vi "Fast_sequence_update_slot.vi"(1 "FPGA Ref":T1, 2 "Points":cluster{string, "data":u64, "data":dbl}, 3 "Inst param":T2) -> (0 "FPGA Ref Out":T1)   [LabVIEW 2013]
uses:
  fpga-bitfile-ref.ctl
  sequence slot/slot-use.ctl
  sequence slot/triggers.ctl
  sequence slot/DAC.ctl
  sequence slot/DAC_fastseq-offset.ctl
  sequence slot/timing.ctl
  sequence slot/jump.ctl
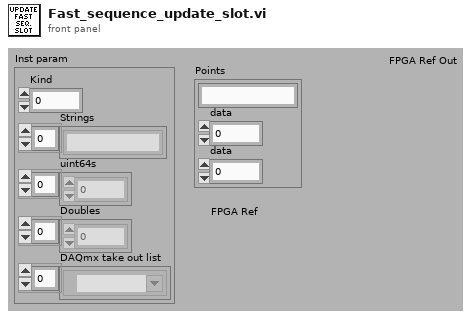
[diagram p1: front panel]
types:
  T1 = typedef "fpga-bitfile-ref.ctl" = refnum<k20>
  T2 = cluster{"Kind":u16, "Strings":string[], "uint64s":u64[], "Doubles":dbl[], "DAQmx take out list":refnum<k21>[]}
  T3 = typedef "slot-use.ctl" = enum8{"DAC", "timing", "triggers", "jump"}
  T4 = typedef "triggers.ctl" = cluster{"triggers":cluster{"1":bool, "2":bool, "3":bool, "4":bool}, "stop":bool}
  T5 = typedef "DAC.ctl" = cluster{"FastChanNum":u8, "DAC offset":T6}
  T6 = typedef "DAC_fastseq-offset.ctl" = sgl
  T7 = typedef "timing.ctl" = sgl
  T8 = typedef "jump.ctl" = u16
  T9 = cluster{"use":T3, "Triggers":T4, "DAC":T5, "timing":T7, "slot#":T8}
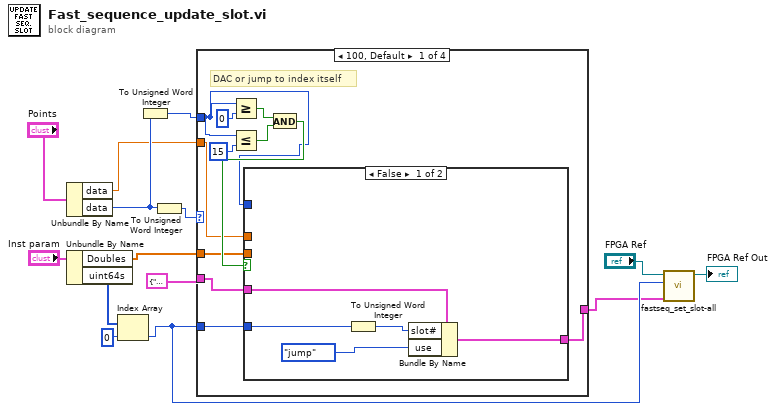
[diagram p0: block diagram]
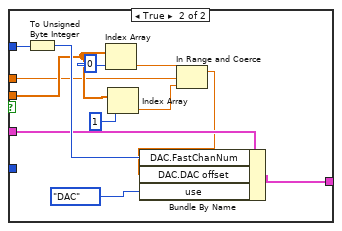
[diagram p2: hidden frame]
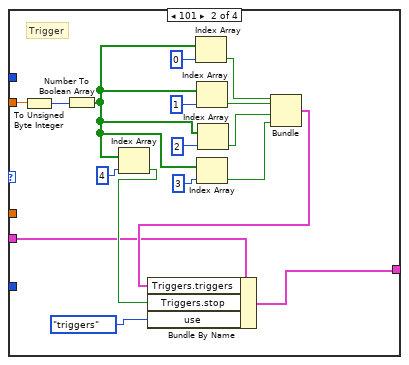
[diagram p3: hidden frame]
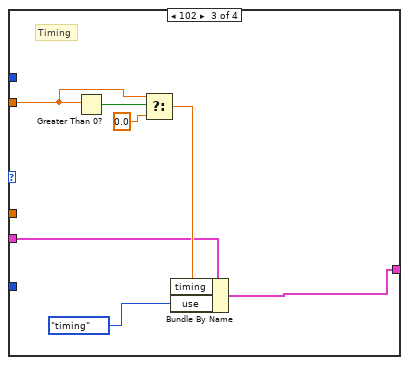
[diagram p4: hidden frame]
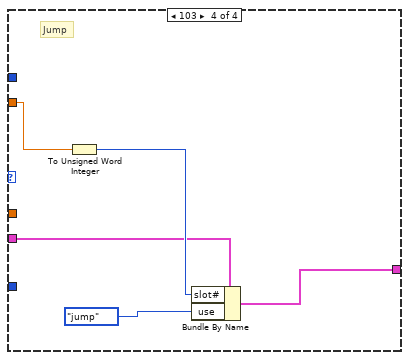
[diagram p5: hidden frame]
diagram:
  n1 = Unbundle By Name("Points") -> ("data"=w11:dbl, "data"=w12:u64)
  n2 = Unbundle By Name("Inst param") -> ("Doubles"=w8:dbl[], "uint64s"=w7:u64[])
  n3 = Index Array(array=w7, index=0) -> (element=w5:u64)
  n4 = To Unsigned Word Integer(number=w12) -> (unsigned 16bit integer=w1:u16)
  n5 = To Unsigned Word Integer(number=w12) -> (unsigned 16bit integer=w13:u16)
  n6 = case shown="100, Default" w13 {
    tunnel: w1 -> [w17 _ _ _]
    tunnel: T9 {"use"=enum."DAC", "Triggers"={"triggers"={"1"=FALSE, "2"=FALSE, "3"=FALSE, "4"=FALSE}, "stop"=FALSE}, "DAC"={"FastChanNum"=0, "DAC offset"=0.0}, "timing"=0.0, "slot#"=0} ("slot 0") -> [w20 w44 w61 w68]
    tunnel: w11 -> [w19 w59 w64 w70]
    tunnel: w8 -> [w18 _ _ _]
    tunnel: [w16 w43 w60 w67] -> w4
    tunnel: w5 -> [w15 _ _ _]
    frame 100, Default {
      # "DAC or jump to index itself"
      n7 = Greater Or Equal?(x=w17, y=0) -> (x >= y?=w25:bool)
      n8 = Less Or Equal?(x=w17, y=15) -> (x <= y?=w24:bool)
      n9 = And(x=w25, y=w24) -> (x .and. y?=w21:bool)
      n10 = case shown="False" w21 {
        tunnel: w20 -> [w28 w37]
        tunnel: w17 -> [_ w42]
        tunnel: w19 -> [_ w32]
        tunnel: w18 -> [_ w33]
        tunnel: [w27 w36] -> w16
        tunnel: w15 -> [w26 _]
        frame False {
          n11 = To Unsigned Word Integer(number=w26) -> (unsigned 16bit integer=w29:u16)
          n12 = Bundle By Name(cluster=w28, "slot#"=w29, "use"=slot-use."jump") -> (w27:T9)
        }
        frame True {
          n13 = To Unsigned Byte Integer(number=w42) -> (unsigned 8bit integer=w40:u8)
          n14 = Index Array(array=w33, index=0) -> (element=w35:dbl)
          n15 = Index Array(array=w33, index=1) -> (element=w34:dbl)
          n16 = In Range and Coerce(upper limit=w35, x=w32, lower limit=w34) -> (coerced(x)=w31:dbl)  [unwired: 1 out]
          n17 = Bundle By Name(cluster=w37, "DAC.FastChanNum"=w40, "DAC.DAC offset"=w31, "use"=slot-use."DAC") -> (w36:T9)
        }
      }
    }
    frame 101 {
      # "Trigger"
      n18 = To Unsigned Byte Integer(number=w59) -> (unsigned 8bit integer=w58:u8)
      n19 = Number To Boolean Array(number=w58) -> (Boolean array=w50:bool[])
      n20 = Index Array(array=w50, index=4) -> (element=w55:bool)
      n21 = Index Array(array=w50, index=0) -> (element=w49:bool)
      n22 = Index Array(array=w50, index=1) -> (element=w48:bool)
      n23 = Index Array(array=w50, index=3) -> (element=w46:bool)
      n24 = Index Array(array=w50, index=2) -> (element=w47:bool)
      n25 = Bundle(w49, w48, w47, w46) -> (w45:cluster{bool, bool, bool, bool})  [unwired: 1 in]
      n26 = Bundle By Name(cluster=w44, "Triggers.triggers"=w45, "Triggers.stop"=w55, "use"=slot-use."triggers") -> (w43:T9)
    }
    frame 102 {
      # "Timing"
      n27 = Greater Than 0?(x=w64) -> (x > 0?=w65:bool)
      n28 = Select(t=w64, s=w65, f=0.0) -> (s? t:f=w62:dbl)
      n29 = Bundle By Name(cluster=w61, "timing"=w62, "use"=slot-use."timing") -> (w60:T9)
    }
    frame 103 {
      # "Jump"
      n30 = To Unsigned Word Integer(number=w70) -> (unsigned 16bit integer=w69:u16)
      n31 = Bundle By Name(cluster=w68, "slot#"=w69, "use"=slot-use."jump") -> (w67:T9)
    }
  }
  n32 = call "fastseq_set_slot-all.vi"("slot"=w4, "slot number"=w5, "FPGA VI Reference In"="FPGA Ref") -> ("FPGA VI Reference Out"=→"FPGA Ref Out":T1)  [unwired: 8 in]
